vi "Get Projects Opened.vi"(8 "error in":errorcluster) -> (0 "error out":errorcluster, 3 "Current Projects Opened":string[](array[string]))   [LabVIEW 2020, in "ConstantErrorsMaker.lvlib"]
uses:
  ConstantErrorsMaker.lvlib
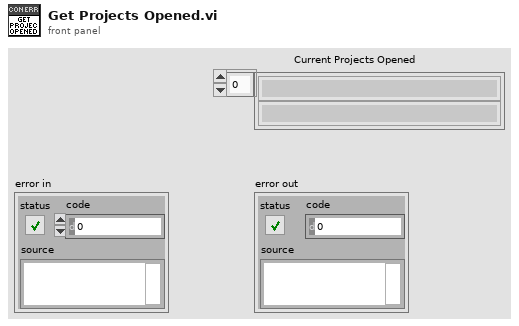
[diagram p1: front panel]
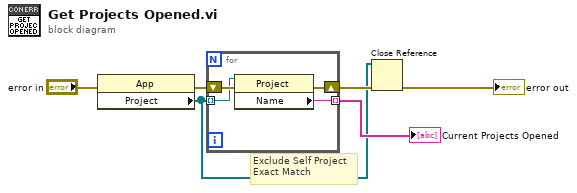
[diagram p0: block diagram]
diagram:
  # "Exclude Self Project\nExact Match"
  n1 = property class="App"(error in="error in") -> (error out=w4:errorcluster, "Project"=w1:refnum<vi>[])  [unwired: 1 in, 1 out]
  n2 = for {
    tunnel: w1 -> [w7] mode=indexing
    tunnel: [w8] -> w2 mode=indexing
    shift-right: [w10] -> w5
    shift-left: w4 -> [w9]
    n3 = property class="Project"(reference=w7, error in=w9) -> (error out=w10:errorcluster, "Name"=w8:string)  [unwired: 1 out]
  }
  "Current Projects Opened" <- w2
  n4 = Close Reference(reference=w1, error in (no error)=w5) -> (error out=→"error out":errorcluster)
